vi "Progress Bar User Interface.vi"(4 "Help String":string, 5 "Global Timeout [mSec] (-1)":i32, 6 "VI":refnum<vi>, 7 "Delay mSec (0)":u32, 8 "error in (no error)":errorcluster, 9 "Explorer Visible? (F)":bool, 10 "Process Events Registration":refnum<event-registration>, 11 "UI Events":T1) -> (0 "error out":errorcluster, 1 "Canceled?":bool)   [LabVIEW 2015, in "Simple Progress Bar.lvlib"]
uses:
  Simple Progress Bar.lvlib
  UI Events.ctl
  Process Events.ctl
  Window States.ctl
  <vilib>/Platform/browser.llb/Open URL in Default Browser (string).vi
panel:
  out "Warnings":string
  out "Item Progression":dbl(slide) scale=0.0..150.0
  out "Job Progression":dbl(slide) scale=0.0..100.0
  out "Item Status":string
  out "Job Status":string
  out "Init":string
  in  "Explore":bool
  in  "Help":bool
  in  "Cancel":bool
  in  "Done":bool
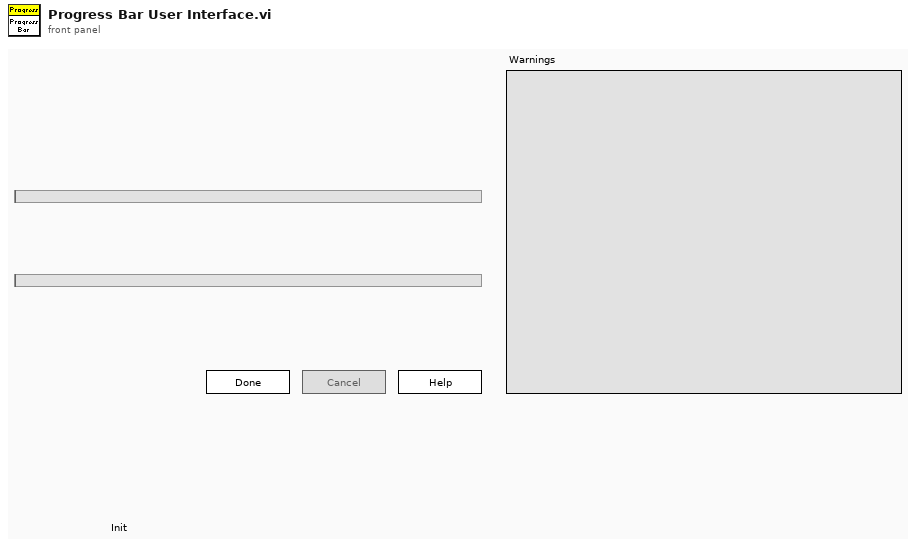
[diagram p1: front panel]
types:
  T1 = typedef "Simple Progress Bar.lvlib/UI Events.ctl" = cluster{"Done":refnum<user-event>, "Cancel":refnum<user-event>, "Explore":refnum<user-event>}
  T2 = enum8{"Enabled", "Disabled", "Disabled and Grayed Out"}
  T3 = enum32{"Invalid", "Standard", "Closed", "Hidden", "Minimized", "Maximized"}
  T4 = typedef "Simple Progress Bar.lvlib/Window States.ctl" = i32
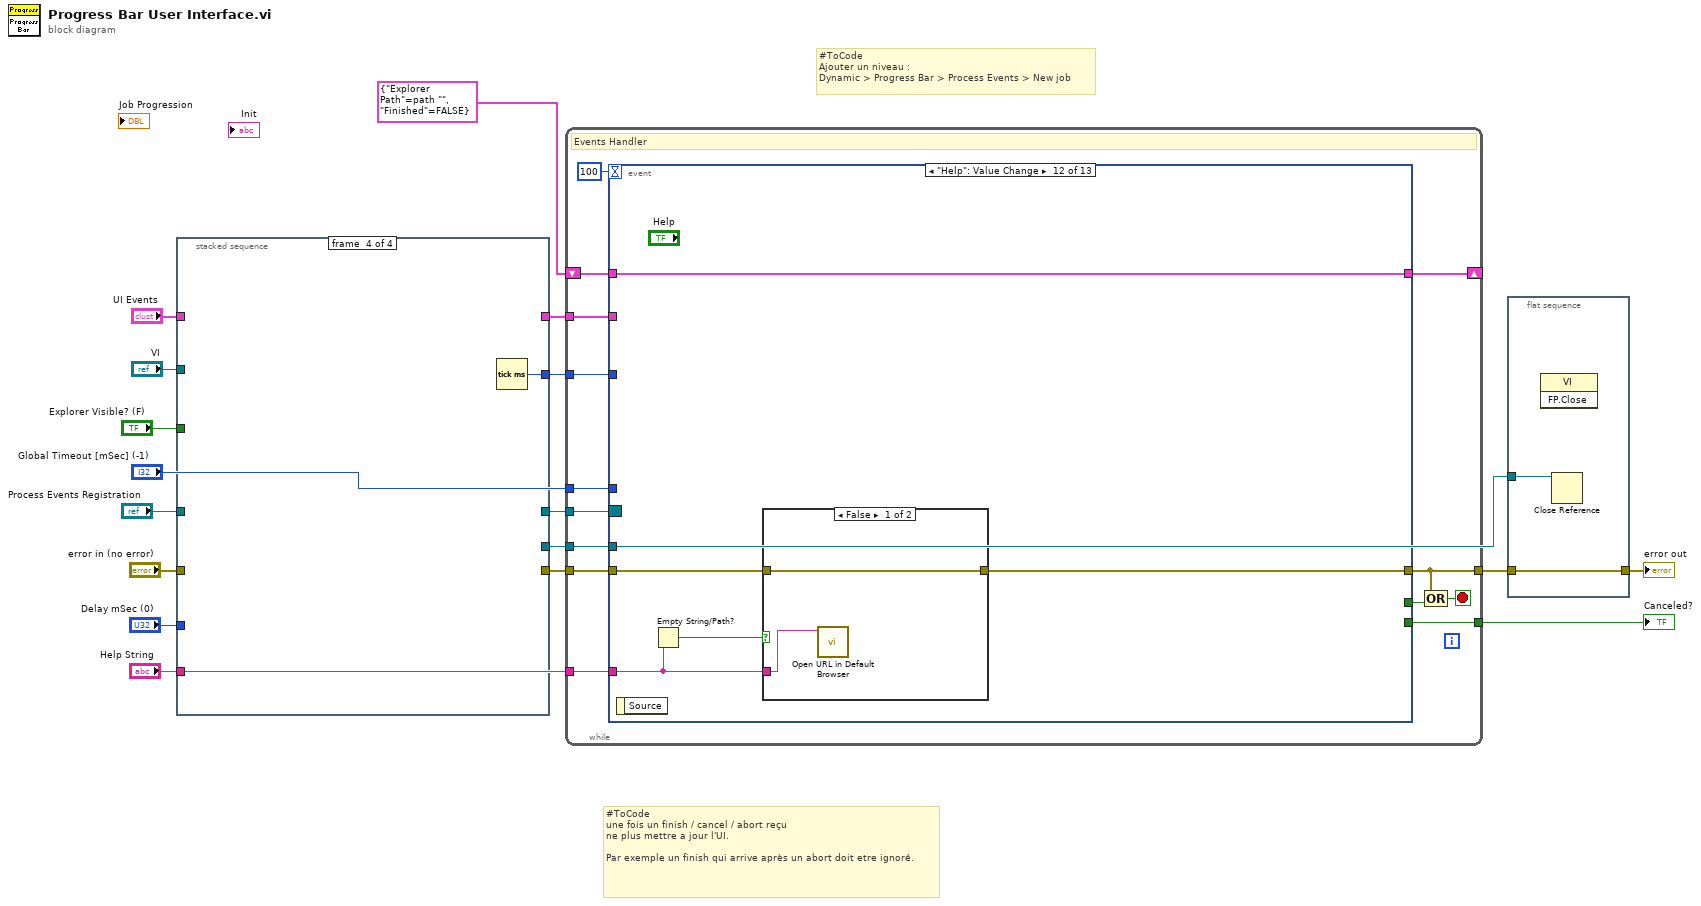
[diagram p0: block diagram]
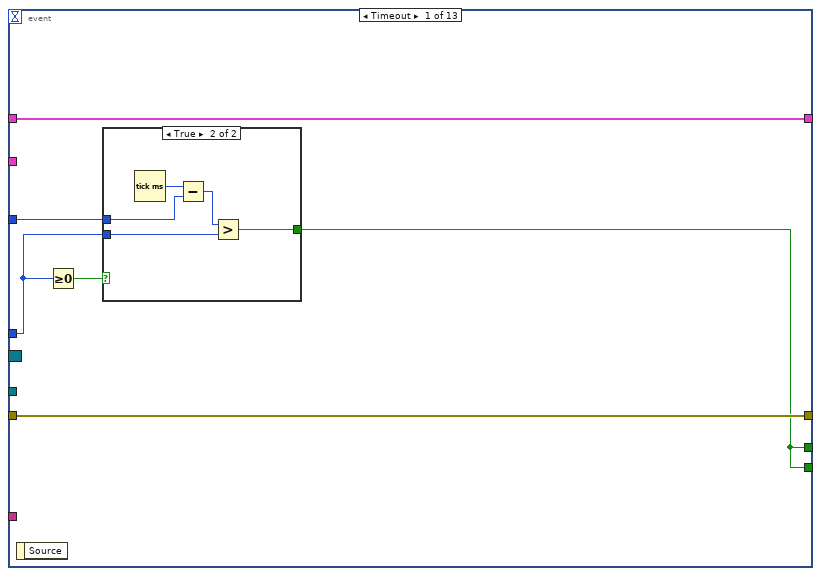
[diagram p2: hidden frame]
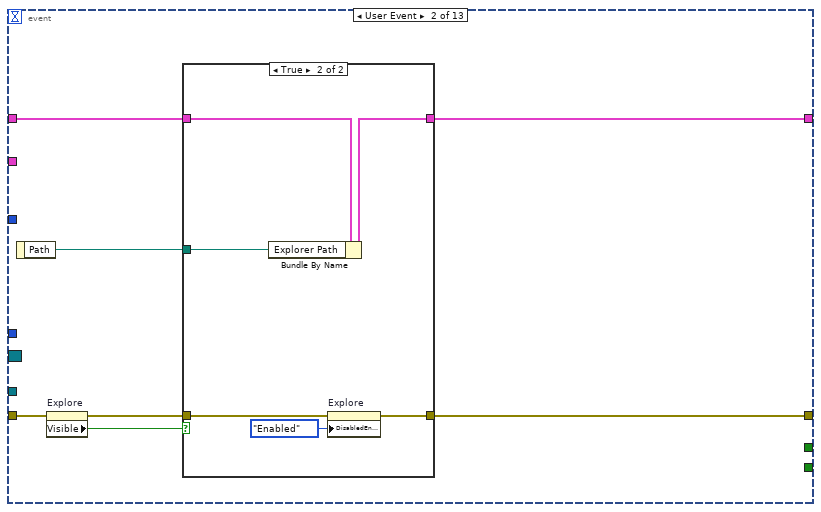
[diagram p4: hidden frame]
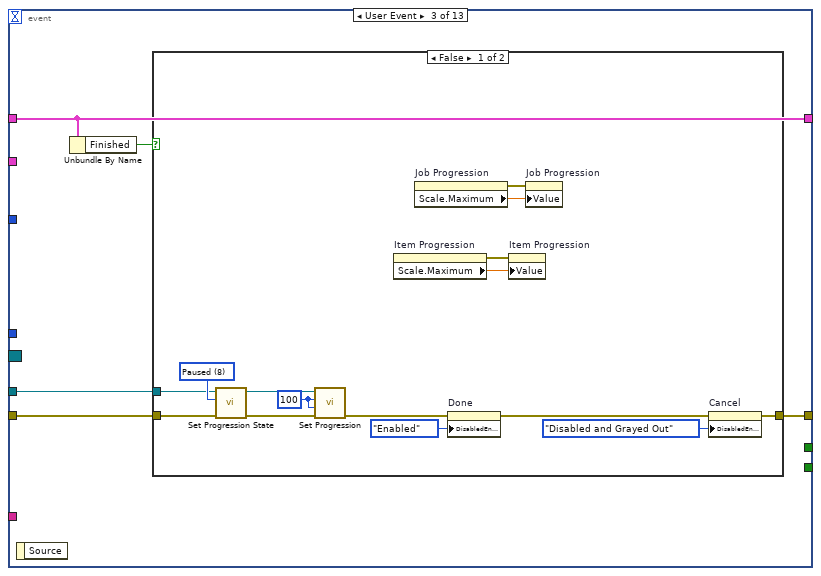
[diagram p6: hidden frame]
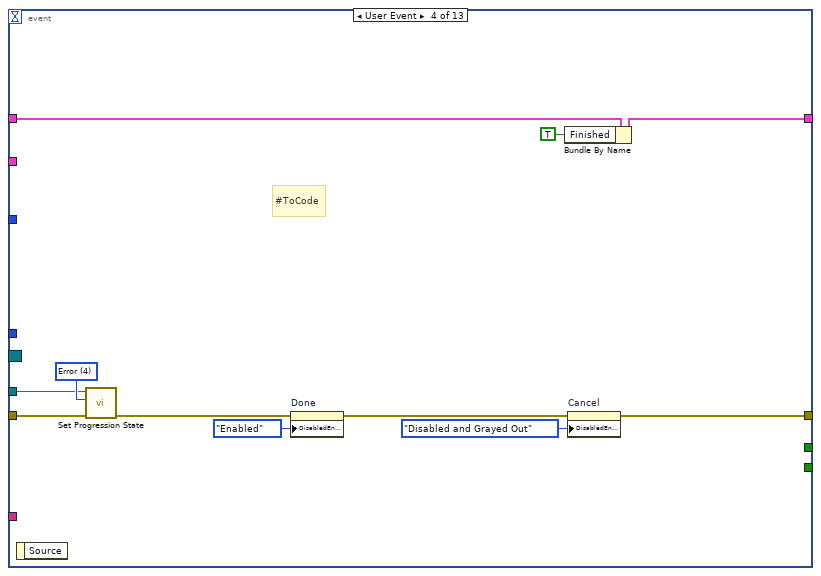
[diagram p8: hidden frame]
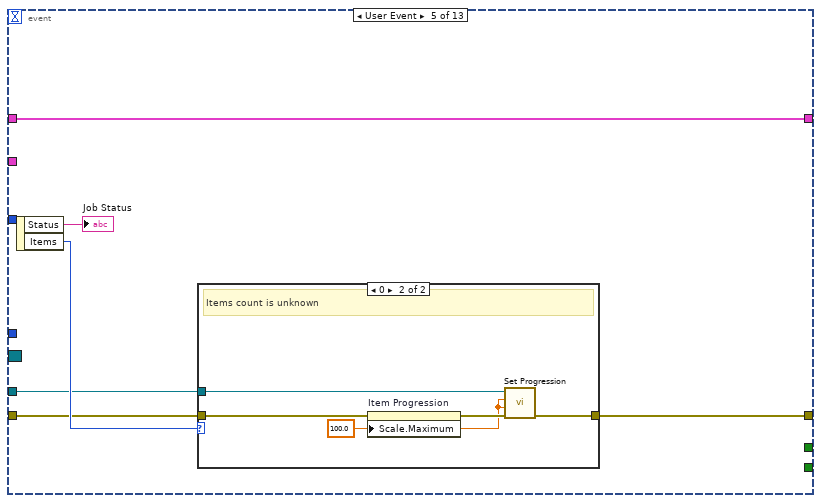
[diagram p9: hidden frame]
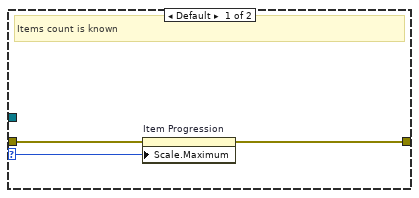
[diagram p10: hidden frame]
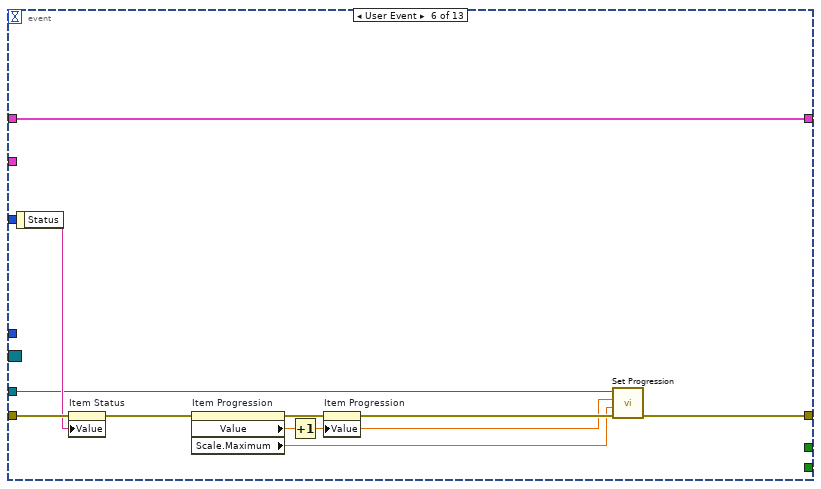
[diagram p11: hidden frame]
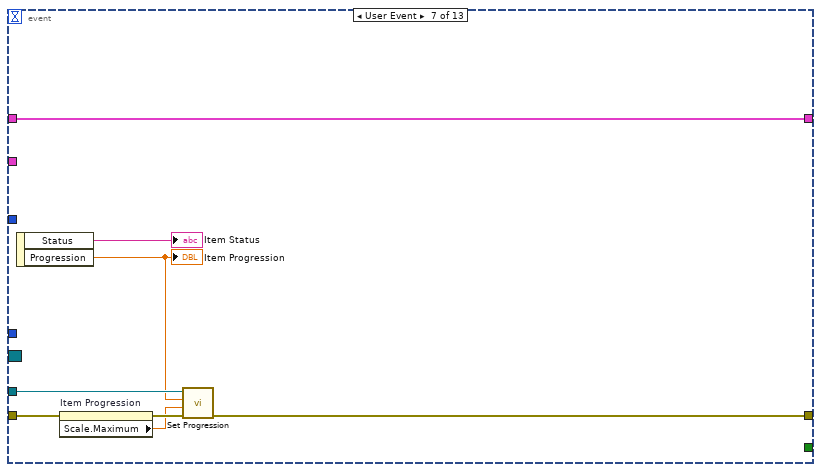
[diagram p12: hidden frame]
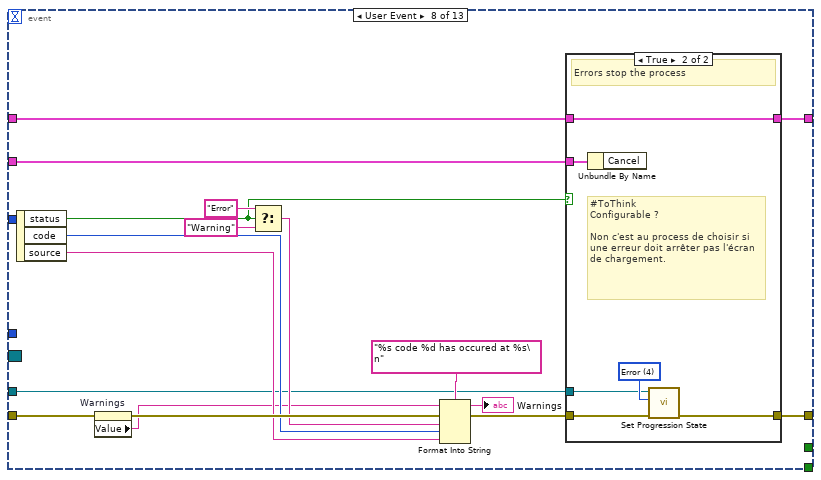
[diagram p13: hidden frame]
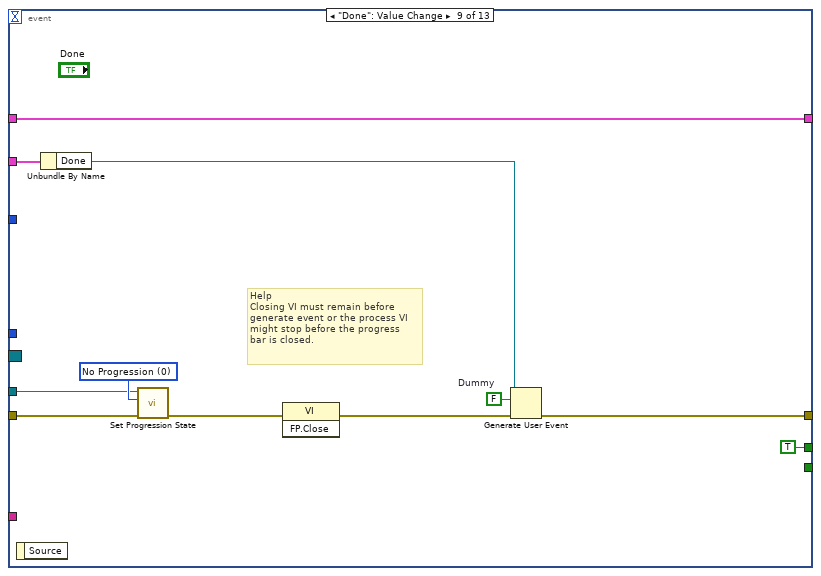
[diagram p15: hidden frame]
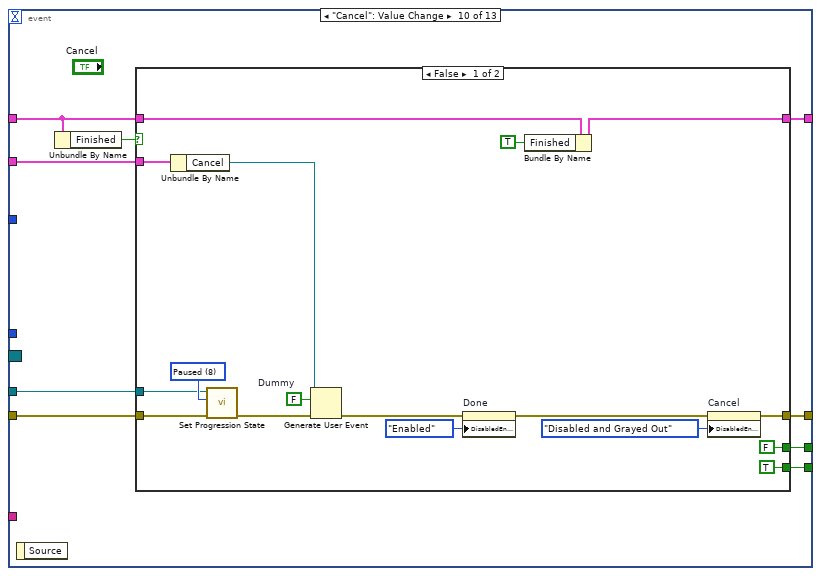
[diagram p16: hidden frame]
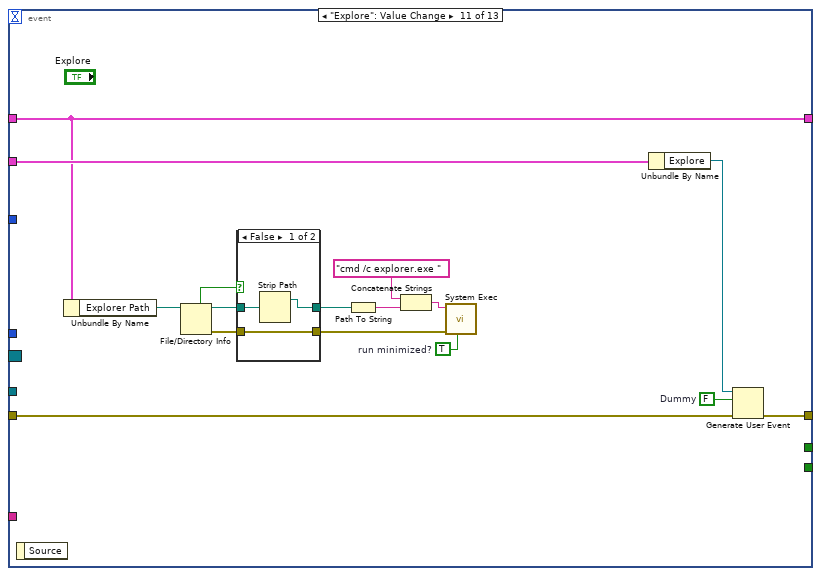
[diagram p18: hidden frame]
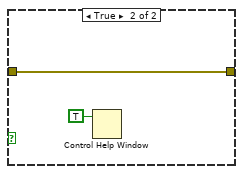
[diagram p20: hidden frame]
diagram:
  # "#ToCode\nune fois un finish / cancel / abort reçu\nne plus mettre a jour l'UI.\n\nPar exemple un finish qui arrive après un abort doit etre ignoré."
  # "#ToCode\nAjouter un niveau :\nDynamic > Progress Bar > Process Events > New job"
  n1 = stacked-sequence {
    tunnel: [_ w22 _ _] -> w16
    tunnel: "error in (no error)" -> [_ w23 _ _]
    tunnel: [_ w27 _ _] -> w14
    tunnel: "UI Events" -> [_ w27 _ _]
    tunnel: [_ w26 _ _] -> w12
    tunnel: "Process Events Registration" -> [_ w26 _ _]
    tunnel: "Explorer Visible? (F)" -> [w18 _ _ _]
    tunnel: "VI" -> [_ w24 _ _]
    tunnel: [_ w21 _ _] -> w7
    tunnel: "Delay mSec (0)" -> [_ _ w36 _]
    tunnel: [_ _ _ w40] -> w3
    tunnel: "Help String" -> [_ _ _ _]
    frame #0 {
      w19 = T2."Disabled and Grayed Out" ("Disabled")
      # "Initialize UI"
      n2 = property on="Explore" class="Bool"("Visible"=w18) -> ()  [unwired: 2 in, 2 out]
      n3 = invoke class="VI" method="Default Vals.Reinit All"() -> ()  [unwired: 3 in, 3 out]
      n4 = property on="Done" class="Bool"("DisabledEnum"=w19) -> ()  [unwired: 2 in, 2 out]
      n5 = property on="Explore" class="Bool"("DisabledEnum"=w19) -> ()  [unwired: 2 in, 2 out]
      n6 = property on="Cancel" class="Bool"("DisabledEnum"=T2."Enabled" ("Disabled")) -> ()  [unwired: 2 in, 2 out]
    }
    frame #1 {
      # "Initialize Data"
      n7 = Not A Number/Path/Refnum?(number/path/refnum=w24) -> (NaN/Path/Refnum?=w25:bool)
      n8 = case shown="False" w25 {
        tunnel: w24 -> [w34 _]
        tunnel: w23 -> [w33 w35]
        tunnel: [w30 w35] -> w22
        tunnel: [w29 _] -> w21
        frame False {
          w28 = T4 2 items=["No Progression"=0, "Indeterminated"=1, "Normal"=2, "Error"=4, "Paused"=8] ("Progression States")
          n9 = call "Find Window Reference.vi"("error in (no error)"=w33, "VI Refnum"=w34) -> ("error out"=w32:errorcluster, "Window Handle"=w31:refnum<k24>)  [unwired: 8 in]
          n10 = call "Set Progression State.vi"("error in (no error)"=w32, "Progression States"=w28, "Window Handle"=w31) -> ("error out"=w30:errorcluster, "Window Handle out"=w29:refnum<k24>)  [unwired: 7 in]
        }
        frame True {
        }
      }
    }
    frame #2 {
      # "Help\nThe interface must be displayed \nafter it has been configured and\ninitialized."
      # "Display interface"
      n11 = flat-sequence {
        tunnel: w36 -> [w37]
        frame #0 {
          n12 = Wait (ms)(milliseconds to wait=w37) -> ()  [unwired: 1 out]
        }
        frame #1 {
          n13 = invoke class="VI" method="FP.Open"("Activate"=TRUE ("Activate?"), "State"=T3."Standard") -> ()  [unwired: 3 in, 5 out]
        }
      }
    }
    frame #3 {
      n14 = Tick Count (ms)() -> (millisecond timer value=w40:u32)
    }
  }
  n15 = while {
    tunnel: w16 -> [w54]
    tunnel: [w51] -> w5
    tunnel: [w53] -> w17
    tunnel: w14 -> [w48]
    tunnel: w12 -> [w47]
    shift-right: [w45] -> _
    shift-left: cluster{"Explorer Path":path, "Finished":bool} {"Explorer Path"=path "", "Finished"=FALSE} -> [w46]
    tunnel: w7 -> [w44]
    tunnel: w3 -> [w43]
    tunnel: "Global Timeout [mSec] (-1)" -> [w42]
    tunnel: "Help String" -> [w41]
    stop <- w49 stop-if-true
    # "Events Handler"
    n16 = event shown="[11] \"Help\": Value Change" {
      selector: w47 -> [_ _ _ _ _ _ _ _ _ _ _ _ _]
      dyn-events: _ -> [_ _ _ _ _ _ _ _ _ _ _ _ _]
      timeout: 100 -> [_ _ _ _ _ _ _ _ _ _ _ _ _]
      tunnel: [w55 _ _ _ _ _ _ _ TRUE ("Exit?") w189 _ _ w245] -> w50
      tunnel: [w60 w70 w84 w106 w114 w127 w142 w150 w180 w185 w223 w231 w240] -> w51
      tunnel: w54 -> [w60 w72 w85 w103 w115 w134 w139 w162 w173 w187 w224 w232 w241]
      tunnel: [w55 _ _ _ _ _ _ _ _ w190 _ _ w243] -> w53
      tunnel: w48 -> [_ _ _ _ _ _ _ w152 w179 w188 w221 _ _]
      tunnel: w46 -> [w59 w69 w83 w112 w118 w137 w145 w148 w176 w184 w220 w235 w242]
      tunnel: [w59 w68 w83 w111 w118 w137 w145 w147 w176 w186 w220 w235 w242] -> w45
      tunnel: w44 -> [_ _ w81 w104 w113 w130 w143 w146 w174 w182 _ _ _]
      tunnel: w43 -> [w58 _ _ _ _ _ _ _ _ _ _ _ _]
      tunnel: w42 -> [w56 _ _ _ _ _ _ _ _ _ _ _ _]
      tunnel: w41 -> [_ _ _ _ _ _ _ _ _ _ _ w233 _]
      event Timeout {
        n17 = event-data() -> ()  [unwired: 1 in, 1 out]
        n18 = Greater Or Equal To 0?(x=w56) -> (x >= 0?=w57:bool)
        n19 = case shown="True" w57 {
          tunnel: w58 -> [_ w64]
          tunnel: w56 -> [_ w62]
          tunnel: [_ w61] -> w55
          frame False {
            # "Global Timeout is disabled"
          }
          frame True {
            n20 = Tick Count (ms)() -> (millisecond timer value=w65:u32)
            n21 = Subtract(x=w65, y=w64) -> (x-y=w63:u32)
            n22 = Greater?(x=w63, y=w62) -> (0:w61:bool)
          }
        }
      }
      event User Event {
        n23 = event-data() -> ("Path"=w66:path)  [unwired: 1 in]
        n24 = property on="Explore" class="Bool"(error in=w72) -> (error out=w71:errorcluster, "Visible"=w67:bool)  [unwired: 1 in, 1 out]
        n25 = case shown="True" w67 {
          tunnel: w71 -> [w73 w80]
          tunnel: [w73 w79] -> w70
          tunnel: w69 -> [w74 w78]
          tunnel: [w74 w76] -> w68
          tunnel: w66 -> [_ w75]
          frame False {
          }
          frame True {
            n26 = Bundle By Name(cluster=w78, "Explorer Path"=w75) -> (w76:cluster{"Explorer Path":path, "Finished":bool})
            n27 = property on="Explore" class="Bool"(error in=w80, "DisabledEnum"=T2."Enabled" ("Disabled")) -> (error out=w79:errorcluster)  [unwired: 1 in, 1 out]
          }
        }
      }
      event User Event {
        n28 = event-data() -> ()  [unwired: 1 in, 1 out]
        n29 = Unbundle By Name(w83) -> ("Finished"=w82:bool)
        n30 = case shown="False" w82 {
          tunnel: w85 -> [w91 w101]
          tunnel: [w99 w101] -> w84
          tunnel: w81 -> [w90 _]
          frame False {
            w86 = u64 100 ("Current Value")
            w92 = T4 8 items=["No Progression"=0, "Indeterminated"=1, "Normal"=2, "Error"=4, "Paused"=8] ("Progression States")
            n31 = call "Set Progression State.vi"("error in (no error)"=w91, "Progression States"=w92, "Window Handle"=w90) -> ("error out"=w89:errorcluster, "Window Handle out"=w88:refnum<k24>)  [unwired: 7 in]
            n32 = call "Set Progression.vi"("error in (no error)"=w89, "Maximum Value (100)"=w86, "Current Value"=w86, "Window Handle"=w88) -> ("error out"=w87:errorcluster)  [unwired: 6 in, 1 out]
            n33 = property on="Item Progression" class="Slide (strict)"() -> (error out=w93:errorcluster, "Scale.Maximum"=w94:dbl)  [unwired: 2 in, 1 out]
            n34 = property on="Job Progression" class="Slide (strict)"() -> (error out=w96:errorcluster, "Scale.Maximum"=w95:dbl)  [unwired: 2 in, 1 out]
            n35 = property on="Done" class="Bool"(error in=w87, "DisabledEnum"=T2."Enabled" ("Disabled")) -> (error out=w100:errorcluster)  [unwired: 1 in, 1 out]
            n36 = property on="Item Progression" class="Slide (strict)"(error in=w93, "Value"=w94) -> ()  [unwired: 1 in, 2 out]
            n37 = property on="Job Progression" class="Slide (strict)"(error in=w96, "Value"=w95) -> ()  [unwired: 1 in, 2 out]
            n38 = property on="Cancel" class="Bool"(error in=w100, "DisabledEnum"=T2."Disabled and Grayed Out" ("Disabled")) -> (error out=w99:errorcluster)  [unwired: 1 in, 1 out]
          }
          frame True {
          }
        }
      }
      event User Event {
        w105 = T4 4 items=["No Progression"=0, "Indeterminated"=1, "Normal"=2, "Error"=4, "Paused"=8] ("Progression States")
        # "#ToCode"
        n39 = event-data() -> ()  [unwired: 1 in, 1 out]
        n40 = call "Set Progression State.vi"("error in (no error)"=w103, "Progression States"=w105, "Window Handle"=w104) -> ("error out"=w102:errorcluster)  [unwired: 7 in, 1 out]
        n41 = property on="Done" class="Bool"(error in=w102, "DisabledEnum"=T2."Enabled" ("Disabled")) -> (error out=w109:errorcluster)  [unwired: 1 in, 1 out]
        n42 = Bundle By Name(cluster=w112, "Finished"=TRUE) -> (w111:cluster{"Explorer Path":path, "Finished":bool})
        n43 = property on="Cancel" class="Bool"(error in=w109, "DisabledEnum"=T2."Disabled and Grayed Out" ("Disabled")) -> (error out=w106:errorcluster)  [unwired: 1 in, 1 out]
      }
      event User Event {
        n44 = event-data() -> ("Status"=→"Job Status":string, "Items"=w116:i32)  [unwired: 1 in]
        n45 = case shown="0" w116 {
          selector: w116 -> [w120 _]
          tunnel: w115 -> [w121 w126]
          tunnel: [w119 w124] -> w114
          tunnel: w113 -> [_ w123]
          frame Default {
            # "Items count is known"
            n46 = property on="Item Progression" class="Slide (strict)"(error in=w121, "Scale.Maximum"=w120) -> (error out=w119:errorcluster)  [unwired: 1 in, 1 out]
          }
          frame 0 {
            w122 = 100.0 ("Scale.Range:Maximum")
            # "Items count is unknown"
            n47 = property on="Item Progression" class="Slide (strict)"(error in=w126, "Scale.Maximum"=w122) -> (error out=w125:errorcluster)  [unwired: 1 in, 1 out]
            n48 = call "Set Progression.vi"("error in (no error)"=w125, "Maximum Value (100)"=w122, "Current Value"=w122, "Window Handle"=w123) -> ("error out"=w124:errorcluster)  [unwired: 6 in, 1 out]
          }
        }
      }
      event User Event {
        n49 = event-data() -> ("Status"=w132:string)  [unwired: 1 in]
        n50 = property on="Item Status" class="Str"(error in=w134, "Value"=w132) -> (error out=w133:errorcluster)  [unwired: 1 in, 1 out]
        n51 = property on="Item Progression" class="Slide (strict)"(error in=w133) -> (error out=w136:errorcluster, "Value"=w135:dbl, "Scale.Maximum"=w129:dbl)  [unwired: 1 in, 1 out]
        n52 = Increment(x=w135) -> (x+1=w128:dbl)
        n53 = property on="Item Progression" class="Slide (strict)"(error in=w136, "Value"=w128) -> (error out=w131:errorcluster)  [unwired: 1 in, 1 out]
        n54 = call "Set Progression.vi"("error in (no error)"=w131, "Maximum Value (100)"=w129, "Current Value"=w128, "Window Handle"=w130) -> ("error out"=w127:errorcluster)  [unwired: 6 in, 1 out]
      }
      event User Event {
        n55 = event-data() -> ("Status"=→"Item Status":string, "Progression"=w138:dbl)  [unwired: 1 in]
        "Item Progression" <- w138
        n56 = property on="Item Progression" class="Slide (strict)"(error in=w139) -> (error out=w141:errorcluster, "Scale.Maximum"=w140:dbl)  [unwired: 1 in, 1 out]
        n57 = call "Set Progression.vi"("error in (no error)"=w141, "Maximum Value (100)"=w140, "Current Value"=w138, "Window Handle"=w143) -> ("error out"=w142:errorcluster)  [unwired: 6 in, 1 out]
      }
      event User Event {
        n58 = event-data() -> ("status"=w149:bool, "code"=w160:i32, "source"=w159:string)  [unwired: 1 in]
        n59 = property on="Warnings" class="Str"(error in=w162) -> (error out=w161:errorcluster, "Value"=w153:string)  [unwired: 1 in, 1 out]
        n60 = Select(t="Error", s=w149, f="Warning") -> (s? t:f=w156:string)
        n61 = Format Into String(format string="%s code %d has occured at %s\n", initial string=w153, error in=w161, w156, w160, w159) -> (resulting string=→"Warnings":string, error out=w151:errorcluster)
        n62 = case shown="True" w149 {
          tunnel: w152 -> [_ w170]
          tunnel: w151 -> [w164 w167]
          tunnel: [w164 w166] -> w150
          tunnel: w148 -> [w163 w169]
          tunnel: [w163 w169] -> w147
          tunnel: w146 -> [_ w165]
          frame False {
            # "Warnings don't stop the process"
          }
          frame True {
            w168 = T4 4 items=["No Progression"=0, "Indeterminated"=1, "Normal"=2, "Error"=4, "Paused"=8] ("Progression States")
            # "#ToThink\nConfigurable ?\n\nNon c'est au process de choisir si une erreur doit arrêter pas l'écran de chargement."
            # "Errors stop the process"
            n63 = Unbundle By Name(w170) -> ()  [unwired: 1 out]
            n64 = call "Set Progression State.vi"("error in (no error)"=w167, "Progression States"=w168, "Window Handle"=w165) -> ("error out"=w166:errorcluster)  [unwired: 7 in, 1 out]
          }
        }
      }
      event "Done": Value Change {
        w175 = T4 0 items=["No Progression"=0, "Indeterminated"=1, "Normal"=2, "Error"=4, "Paused"=8] ("Progression States")
        w177 = FALSE  # Dummy
        # "Help\nClosing VI must remain before \ngenerate event or the process VI \nmight stop before the progress \nbar is closed."
        n65 = event-data() -> ()  [unwired: 1 in, 1 out]
        n66 = Unbundle By Name(w179) -> ("Done"=w178:refnum<user-event>)
        n67 = call "Set Progression State.vi"("error in (no error)"=w173, "Progression States"=w175, "Window Handle"=w174) -> ("error out"=w172:errorcluster)  [unwired: 7 in, 1 out]
        n68 = invoke class="VI" method="FP.Close"(error in=w172) -> (error out=w171:errorcluster)  [unwired: 2 in, 2 out]
        n69 = Generate User Event(user event=w178, event data cluster=w177, error in=w171) -> (error out=w180:errorcluster)  [unwired: 1 in, 1 out]
      }
      event "Cancel": Value Change {
        n70 = event-data() -> ()  [unwired: 1 in, 1 out]
        n71 = Unbundle By Name(w184) -> ("Finished"=w183:bool)
        n72 = case shown="False" w183 {
          tunnel: [TRUE ("Canceled?") _] -> w190
          tunnel: [FALSE ("Exit?") _] -> w189
          tunnel: w188 -> [w204 _]
          tunnel: w187 -> [w192 w208]
          tunnel: [w202 w209] -> w186
          tunnel: [w196 w208] -> w185
          tunnel: w184 -> [w195 w209]
          tunnel: w182 -> [w193 _]
          frame False {
            w194 = T4 8 items=["No Progression"=0, "Indeterminated"=1, "Normal"=2, "Error"=4, "Paused"=8] ("Progression States")
            w205 = FALSE  # Dummy
            n73 = Unbundle By Name(w204) -> ("Cancel"=w203:refnum<user-event>)
            n74 = call "Set Progression State.vi"("error in (no error)"=w192, "Progression States"=w194, "Window Handle"=w193) -> ("error out"=w191:errorcluster)  [unwired: 7 in, 1 out]
            n75 = Generate User Event(user event=w203, event data cluster=w205, error in=w191) -> (error out=w197:errorcluster)  [unwired: 1 in, 1 out]
            n76 = property on="Done" class="Bool"(error in=w197, "DisabledEnum"=T2."Enabled" ("Disabled")) -> (error out=w200:errorcluster)  [unwired: 1 in, 1 out]
            n77 = Bundle By Name(cluster=w195, "Finished"=TRUE) -> (w202:cluster{"Explorer Path":path, "Finished":bool})
            n78 = property on="Cancel" class="Bool"(error in=w200, "DisabledEnum"=T2."Disabled and Grayed Out" ("Disabled")) -> (error out=w196:errorcluster)  [unwired: 1 in, 1 out]
          }
          frame True {
          }
        }
      }
      event "Explore": Value Change {
        w212 = TRUE  # run minimized?
        w225 = FALSE  # Dummy
        n79 = event-data() -> ()  [unwired: 1 in, 1 out]
        n80 = Unbundle By Name(w220) -> ("Explorer Path"=w219:path)
        n81 = File/Directory Info(path=w219) -> (path out=w217:path, directory=w218:bool, error out=w216:errorcluster)  [unwired: 1 in, 4 out]
        n82 = case shown="False" w218 {
          tunnel: w217 -> [w228 w230]
          tunnel: [w227 w230] -> w210
          tunnel: [w226 w229] -> w211
          tunnel: w216 -> [w226 w229]
          frame False {
            n83 = Strip Path(path=w228) -> (stripped path=w227:path)  [unwired: 1 out]
          }
          frame True {
          }
        }
        n84 = Path To String(path=w210) -> (string=w214:string)
        n85 = Concatenate Strings("cmd /c explorer.exe ", w214) -> (w213:string)
        n86 = call <vilib>:"System Exec.vi"("run minimized? (F)"=w212, "error in (no error)"=w211, "command line"=w213) -> ()  [unwired: 5 in, 4 out]
        n87 = Unbundle By Name(w221) -> ("Explore"=w222:refnum<user-event>)
        n88 = Generate User Event(user event=w222, event data cluster=w225, error in=w224) -> (error out=w223:errorcluster)  [unwired: 1 in, 1 out]
      }
      event "Help": Value Change {
        n89 = event-data() -> ()  [unwired: 1 in, 1 out]
        n90 = Empty String/Path?(string/path=w233) -> (empty?=w234:bool)
        n91 = case shown="False" w234 {
          tunnel: w233 -> [w237 _]
          tunnel: w232 -> [w236 w238]
          tunnel: [w236 w238] -> w231
          frame False {
            n92 = call-poly <vilib>:"Open URL in Default Browser.vi"("URL"=w237) -> ()  [unwired: 5 in, 2 out]
          }
          frame True {
            n93 = Control Help Window(1:TRUE ("Show")) -> ()  [unwired: 1 in]
          }
        }
      }
      event Panel Close? {
        w243 = FALSE  # Canceled?
        w245 = FALSE  # Exit?
        # "Closing the window don't stop the VI."
        n94 = event-data() -> ()  [unwired: 1 in, 1 out]
        n95 = invoke class="VI" method="FP.Close"(error in=w241) -> (error out=w240:errorcluster)  [unwired: 2 in, 2 out]
        n96 = event-data("Discard?"=TRUE) -> ()  [unwired: 1 in, 1 out]
      }
    }
    n97 = Compound Arithmetic op=OR(w51, w50) -> (w49:bool)
  }
  "Canceled?" <- w17
  n98 = flat-sequence {
    tunnel: w7 -> [w246]
    tunnel: [w247] -> w6
    tunnel: w5 -> [w247]
    frame #0 {
      n99 = invoke class="VI" method="FP.Close"() -> ()  [unwired: 3 in, 3 out]
      n100 = Close Reference(reference=w246) -> ()  [unwired: 1 in, 1 out]
    }
  }
  "error out" <- w6
